vi "Product Selection.vi"(8 "error in (no error)":errorcluster, 10 "Products":i32, 11 "Products Picker in":refnum<class "Products Picker.lvclass">) -> (0 "error out":errorcluster, 3 "Products Picker out":refnum<class "Products Picker.lvclass">)   [LabVIEW 2020, in "Products Picker.lvlib" / "Products Picker.lvclass"]
uses:
  Products Picker.lvclass
  Products Picker.lvclass/Products Picker.ctl
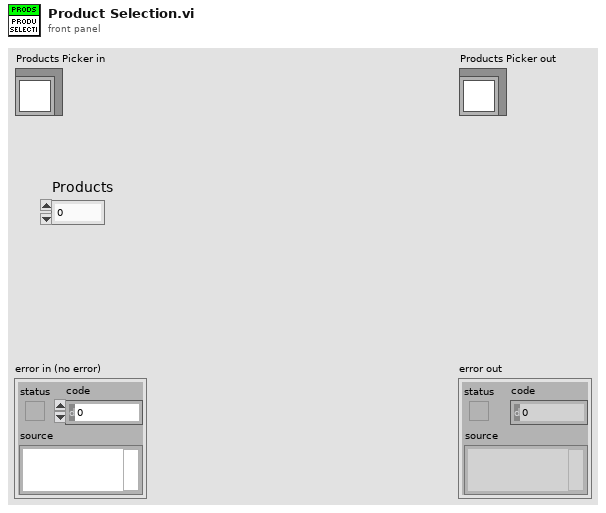
[diagram p1: front panel]
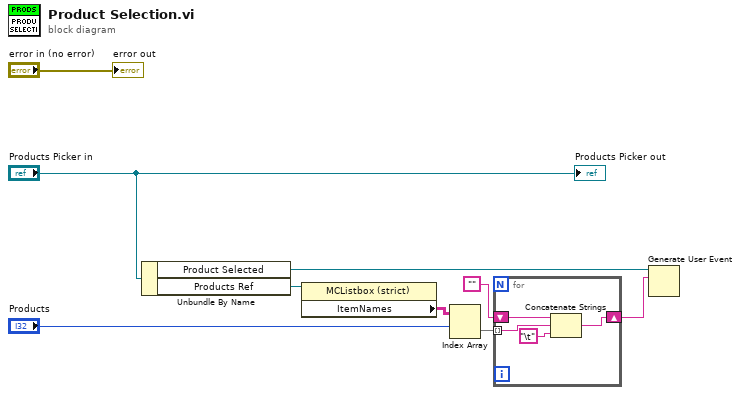
[diagram p0: block diagram]
diagram:
  n1 = Unbundle By Name("Products Picker in") -> ("Product Selected"=w4:refnum<user-event>, "Products Ref"=w6:refnum<vi>)
  n2 = property class="MCListbox (strict)"(reference=w6) -> ("ItemNames"=w5:string[][])  [unwired: 1 in, 2 out]
  n3 = Index Array(array=w5, index (row)="Products") -> (element=w3:string[])  [unwired: 1 in]
  n4 = for {
    tunnel: w3 -> [w13] mode=indexing
    shift-right: [w12] -> w1
    shift-left: "" -> [w11]
    n5 = Concatenate Strings(w11, w13, "\t") -> (w12:string)
  }
  n6 = Generate User Event(user event=w4, event data cluster=w1) -> ()  [unwired: 2 in, 2 out]
  "error out" <- "error in (no error)"
  "Products Picker out" <- "Products Picker in"
